vi "Single Channel output c.vi"(4 "Reset by Enc C":bool, 5 "Reset by hand":bool, 6 "DIR":bool, 7 "Period (Ticks)":u32=2000, 8 "STBY":bool, 9 "ENA":bool, 10 "Duty":fxp<+,32,0>, 11 "I/O Channel":T1={"Encoder C"="ConnectorA/DIO13", "Encoder B"="ConnectorA/DIO12", "Encoder A"="ConnectorA/DIO11", "PWM"="ConnectorA/DIO10", "DIR"="ConnectorA/DIO9", "STBY"="ConnectorA/DIO8", "ENA"="ConnectorA/DIO7"}) -> (1 "C":bool, 2 "JumpBy2Error":i16, 3 "Position":i32)   [LabVIEW 2018]
uses:
  <vilib>/rvi/eio/common/nirviEmuTemplateMethod_errors.vi
  <vilib>/eio/EIONode/EIONode.xnode
  jmslib.lvlib
  kevLib2010.lvlib
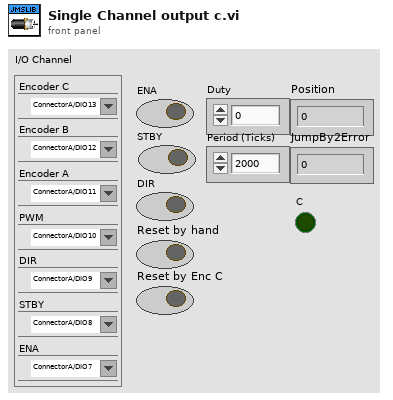
[diagram p1: front panel]
types:
  T1 = cluster{"Encoder C":refnum<k21>, "Encoder B":refnum<k21>, "Encoder A":refnum<k21>, "PWM":refnum<k21>, "DIR":refnum<k21>, "STBY":refnum<k21>, "ENA":refnum<k21>}
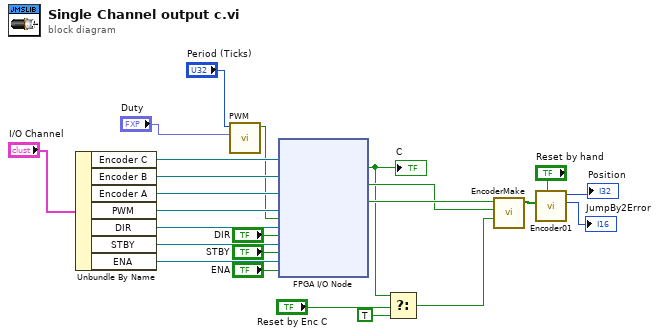
[diagram p0: block diagram]
diagram:
  n1 = Unbundle By Name("I/O Channel") -> ("Encoder C"=w20:refnum<k21>, "Encoder B"=w19:refnum<k21>, "Encoder A"=w18:refnum<k21>, "PWM"=w17:refnum<k21>, "DIR"=w16:refnum<k21>, "STBY"=w15:refnum<k21>, "ENA"=w14:refnum<k21>)
  n2 = call "PWM.vi"("Duty Cycle"="Duty", "Period (Ticks)"="Period (Ticks)") -> ("PWM Out"=w6:bool)  [unwired: 8 in, 1 out]
  n3 = xnode "FPGA I/O Node"("FPGA I/O In"=w20, "FPGA I/O In"=w19, "FPGA I/O In"=w18, "I/O Item"=w6, "FPGA I/O In"=w17, "I/O Item"="DIR", "FPGA I/O In"=w16, "I/O Item"="STBY", "FPGA I/O In"=w15, "I/O Item"="ENA", "FPGA I/O In"=w14) -> ("I/O Item"=w1:bool, "I/O Item"=w3:bool, "I/O Item"=w4:bool)  [unwired: 7 out]
  "C" <- w1
  n4 = Select(t=w1, s="Reset by Enc C", f=TRUE ("C")) -> (s? t:f=w11:bool)
  n5 = call "EncoderMake.vi"("C"=w11, "B"=w3, "A"=w4) -> ("Encoder Array"=w23:bool[])  [unwired: 8 in]
  n6 = call "Encoder01.vi"("ForceReset"="Reset by hand", "Encoder Array"=w23) -> ("JumpBy2Error"=→"JumpBy2Error":i16, "Position"=→"Position":i32)  [unwired: 6 in, 2 out]
